vi "Create_Config.vi"(8 "Error In":errorcluster, 11 "Data":T1) -> (0 "Error Out":errorcluster)   [LabVIEW 2017]
uses:
  data.ctl
  <vilib>/Utility/file.llb/Write Delimited Spreadsheet (string).vi
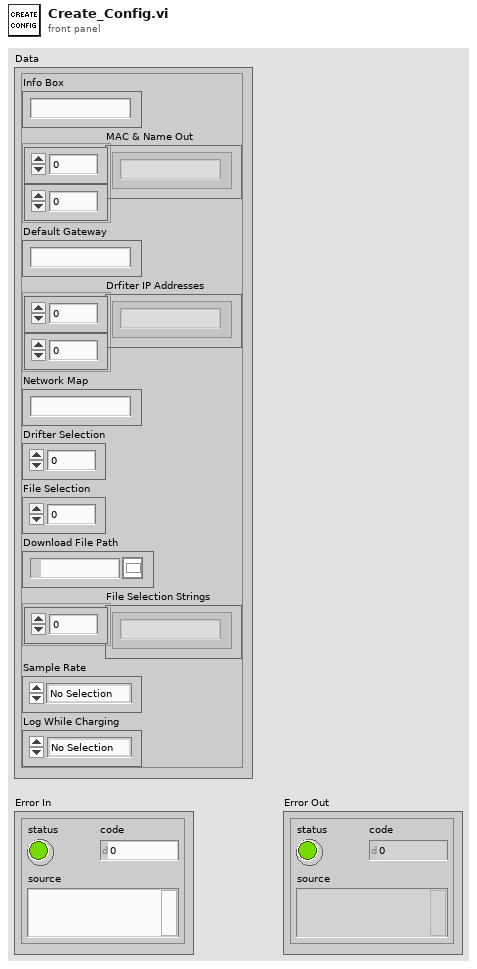
[diagram p1: front panel]
types:
  T1 = typedef "data.ctl" = cluster{"Info Box":string, "MAC & Name Out":string[][], "Default Gateway":string, "Drfiter IP Addresses":string[][], "Network Map":string, "Drifter Selection":i32, "File Selection":i32, "Download File Path":path, "File Selection Strings":string[], "Sample Rate":enum32{"No Selection", " 0.2", " 0.1", " 1", " 2", " 5", " 10"}, "Log While Charging":enum32{"No Selection", " Yes", " No"}}
  T2 = enum32{"No Selection", " 0.2", " 0.1", " 1", " 2", " 5", " 10"}
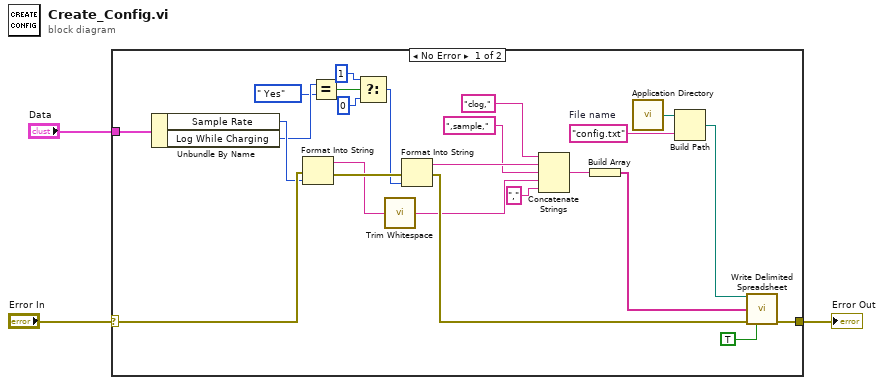
[diagram p0: block diagram]
diagram:
  n1 = case shown="No Error" "Error In" {
    selector: "Error In" -> [w21 w28]
    tunnel: [w23 w28] -> w1
    tunnel: "Data" -> [w22 _]
    frame No Error {
      w27 = "config.txt"  # File name
      n2 = Unbundle By Name(w22) -> ("Sample Rate"=w20:T2, "Log While Charging"=w8:enum32{"No Selection", " Yes", " No"})
      n3 = Format Into String(error in=w21, w20) -> (resulting string=w11:string, error out=w19:errorcluster)  [unwired: 2 in]
      n4 = Equal?(x=w8, y=enum32{"No Selection", " Yes", " No"}." Yes") -> (x = y?=w9:bool)
      n5 = Select(t=i8 1, s=w9, f=i8 0 ("t")) -> (s? t:f=w4:i8)
      n6 = call <vilib>:"Trim Whitespace.vi"("string"=w11) -> ("trimmed string"=w10:string)  [unwired: 1 in]
      n7 = Format Into String(error in=w19, w4) -> (resulting string=w16:string, error out=w18:errorcluster)  [unwired: 2 in]
      n8 = Concatenate Strings("clog,", w16, ",sample," ("element"), w10, "," ("element")) -> (w13:string)
      n9 = Build Array(w13) -> (w12:string[])
      n10 = call <vilib>:"Application Directory.vi"() -> ("Application Directory"=w26:path)
      n11 = Build Path(base path=w26, name or relative path=w27) -> (appended path=w25:path)
      n12 = call-poly <vilib>:"Write Delimited Spreadsheet.vi"("file path (dialog if empty)"=w25, "1D data"=w12, "error in (no error)"=w18, "transpose? (no:F)"=TRUE) -> ("error out"=w23:errorcluster)  [unwired: 10 in, 1 out]
    }
    frame Error {
    }
  }
  "Error Out" <- w1
